vi "ListServerErrors.vi"() -> (2 "Array":string[][](array[string]), 3 "Total Server Errors":i32)   [LabVIEW 2012]
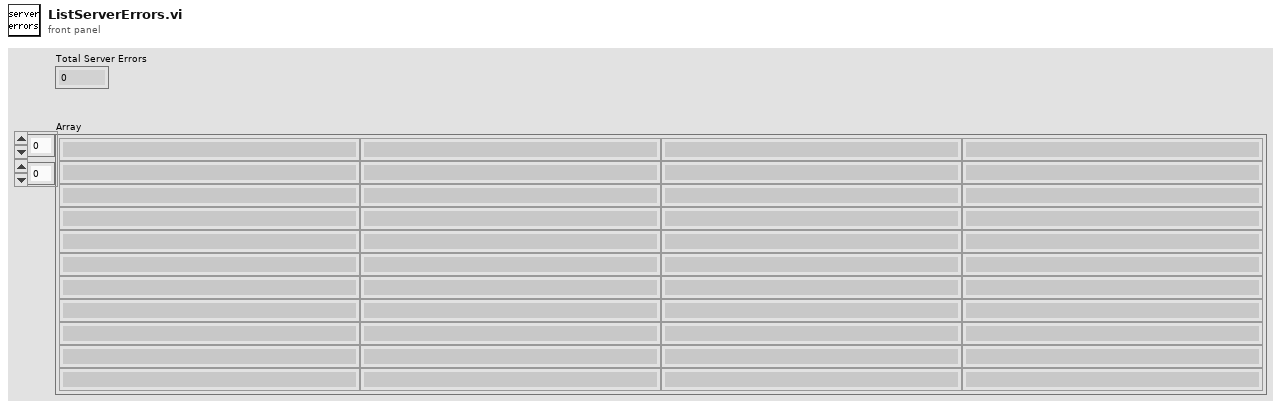
[diagram p1: front panel]
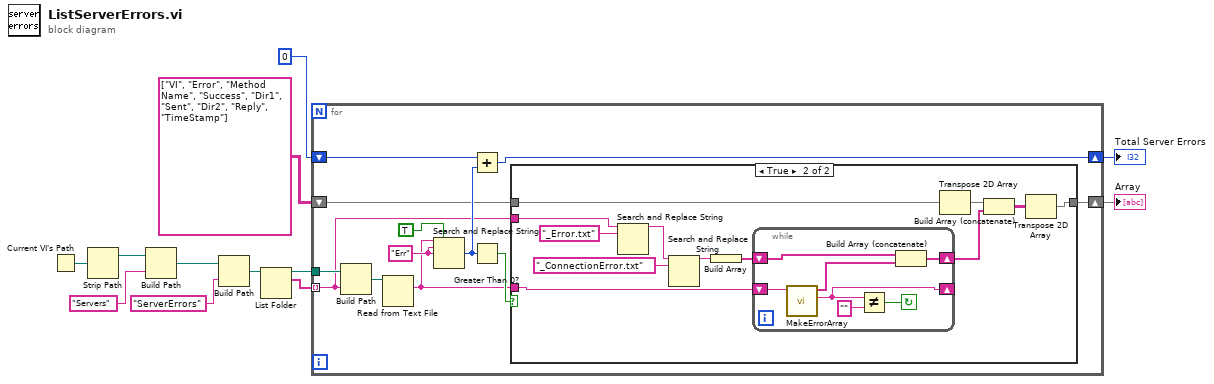
[diagram p0: block diagram]
diagram:
  n1 = Current VI's Path() -> (path=w4:path)
  n2 = Strip Path(path=w4) -> (stripped path=w3:path)  [unwired: 1 out]
  n3 = Build Path(base path=w3, name or relative path="Servers") -> (appended path=w6:path)
  n4 = Build Path(base path=w6, name or relative path="ServerErrors") -> (appended path=w11:path)
  n5 = List Folder(path=w11) -> (path out=w9:path, filenames=w10:string[])  [unwired: 3 in, 2 out]
  n6 = for {
    tunnel: w10 -> [w16] mode=indexing
    tunnel: w9 -> [w24]
    shift-right: [w20] -> w7
    shift-left: 0 ("number of replacements") -> [w21]
    shift-right: [w15] -> w1
    shift-left: string[][] [["VI"], ["Error"], ["Method Name"], ["Success"], ["Dir1"], ["Sent"], ["Dir2"], ["Reply"], ["TimeStamp"]] -> [w14]
    w22 = "Err" ("search string")
    n7 = Build Path(base path=w24, name or relative path=w16) -> (appended path=w23:path)
    n8 = Read from Text File(file (use dialog)=w23) -> (text=w17:string)  [unwired: 3 in, 3 out]
    n9 = Search and Replace String(replace all?=TRUE ("replace all? (F)"), input string=w17, search string=w22, replace string=w22) -> (number of replacements=w18:i32)  [unwired: 4 in, 3 out]
    n10 = Add(x=w21, y=w18) -> (x+y=w20:i32)
    n11 = Greater Than 0?(x=w18) -> (x > 0?=w19:bool)
    n12 = case shown="True" w19 {
      tunnel: w17 -> [_ w37]
      tunnel: w16 -> [_ w33]
      tunnel: [w25 w29] -> w15
      tunnel: w14 -> [w25 w27]
      frame False {
      }
      frame True {
        n13 = Search and Replace String(input string=w33, search string="_Error.txt") -> (result string=w35:string)  [unwired: 6 in, 3 out]
        n14 = Search and Replace String(input string=w35, search string="_ConnectionError.txt") -> (result string=w32:string)  [unwired: 6 in, 3 out]
        n15 = Build Array(w32) -> (w31:string[])
        n16 = while {
          shift-right: [w41] -> _
          shift-left: w37 -> [w44]
          shift-right: [w38] -> w28
          shift-left: w31 -> [w39]
          stop <- w43 continue-if-true
          n17 = call <userlib>:"MakeErrorArray.vi"("In"=w44) -> ("Out"=w41:string, "ErrorArray"=w40:string[])  [unwired: 9 in]
          n18 = Not Equal?(x=w41, y="") -> (x != y?=w43:bool)
          n19 = Build Array (concatenate)(w39, w40) -> (w38:string[])
        }
        n20 = Transpose 2D Array(2D array=w27) -> (transposed array=w26:string[][])
        n21 = Build Array (concatenate)(w26, w28) -> (w30:string[][])
        n22 = Transpose 2D Array(2D array=w30) -> (transposed array=w29:string[][])
      }
    }
  }
  "Total Server Errors" <- w7
  "Array" <- w1
